vi "Open HTTP connection.vi"(7 "remote port":u16=80, 8 "error in (no error)":errorcluster, 9 "password":string, 10 "username":string="kirsch", 11 "Camera address":string="10.0.7.103") -> (0 "error out":errorcluster, 3 "TCP Network Connection out":refnum<k5>)   [LabVIEW 2014]
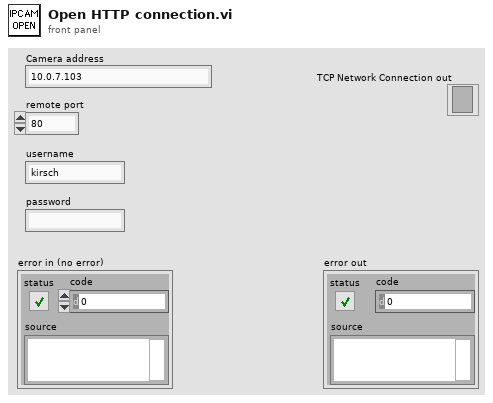
[diagram p1: front panel]
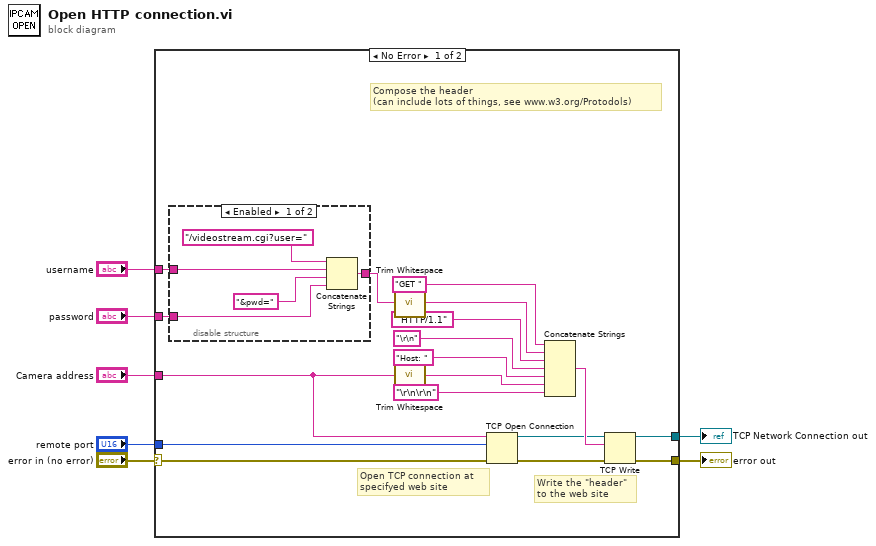
[diagram p0: block diagram]
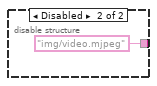
[diagram p2: hidden frame]
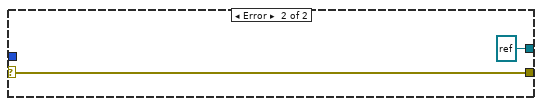
[diagram p3: hidden frame]
diagram:
  n1 = case shown="No Error" "error in (no error)" {
    selector: "error in (no error)" -> [w8 w33]
    tunnel: "username" -> [w25 _]
    tunnel: "password" -> [w24 _]
    tunnel: "Camera address" -> [w20 _]
    tunnel: "remote port" -> [w14 _]
    tunnel: [w13 w33] -> w3
    tunnel: [w12 refnum<k5> refnum ("connection ID")] -> w2
    frame No Error {
      # "Compose the header\n(can include lots of things, see www.w3.org/Protodols)"
      # "Write the \"header\"\nto the web site"
      # "Open TCP connection at\nspecifyed web site"
      n2 = disable-structure shown="Enabled" {
        disable-tunnel: w25 -> [w29 _]
        disable-tunnel: w24 -> [w27 _]
        disable-tunnel: [w26 "img/video.mjpeg" ("string")] -> w9
        frame Enabled {
          n3 = Concatenate Strings("/videostream.cgi?user=" ("Path"), w29, "&pwd=" ("more path"), w27) -> (w26:string)
        }
        frame Disabled {
        }
      }
      n4 = call <vilib>:"Trim Whitespace.vi"("string"=w9) -> ("trimmed string"=w16:string)  [unwired: 1 in]
      n5 = call <vilib>:"Trim Whitespace.vi"("string"=w20) -> ("trimmed string"=w21:string)  [unwired: 1 in]
      n6 = TCP Open Connection(address=w20, remote port or service name=w14, error in (no error)=w8) -> (connection ID=w11:refnum<k5>, error out=w10:errorcluster)  [unwired: 2 in]
      n7 = Concatenate Strings("GET " ("Command"), w16, " HTTP/1.1" ("Command"), "\r\n" ("string"), "Host: " ("Command"), w21, "\r\n\r\n" ("string")) -> (w23:string)
      n8 = TCP Write(connection ID=w11, data in=w23, error in (no error)=w10) -> (connection ID out=w12:refnum<k5>, error out=w13:errorcluster)  [unwired: 1 in, 1 out]
    }
    frame Error {
    }
  }
  "error out" <- w3
  "TCP Network Connection out" <- w2
